vi "Dictionary Open Object Reference__ogtk.vi"(8 "error in (no error)":errorcluster) -> (0 "error out":errorcluster, 3 "Object RefNum":T1)   [LabVIEW 2017]
uses:
  <userlib>/_OpenG.lib/dictionary/dictionary.llb/Dictionary Object RefNum__ogtk.ctl
  <userlib>/_OpenG.lib/dictionary/dictionary.llb/Dictionary Object RefNum - Enum__ogtk.ctl
  <userlib>/_OpenG.lib/dictionary/dictionary.llb/Dictionary Object Data Core Task Enum__ogtk.ctl
panel:
  # "<VI Name>\n\n<VI Description>\n\nPlease visit http://www.OpenG.org to learn about the\nOpen Source LabVIEW software movement.\n\nNOTICE -- YOU MUST LEAVE THIS NOTICE IN PLACE.  PER THE TERMS OF THE LICENSE BELOW, YOU MAY SUBLICENSE THIS SOFTWARE \nIN ANY WAY THAT DOES NOT CONFLICT WITH THIS LICENSE.\n\n### BSD License (http://www.opensource.org/licenses/bsd-license.php) Begin ###\n \nCopyright (c) 2003, Jim Kring <jim@jimkring.com>\n\nAll rights reserved.\n\nRedistribution and use in source and binary forms, with or without modification, are permitted provided that the following conditions are met:\n\n    * Redistributions of source code must retain the above copyright notice, this list of conditions and the following disclaimer.\n    * Redistributions in binary form must reproduce the above copyright notice, this list of conditions and the following disclaimer in the \n       documentation and/or other materials provided with the distribution.\n    * Neither the name of SciWare, James Kring, Inc., nor the names of its contributors may be used to endorse or promote products derived \n       from this software without specific prior written permission.\n\nTHIS SOFTWARE IS PROVIDED BY THE COPYRIGHT HOLDERS AND CONTRIBUTORS \"AS IS\" AND ANY EXPRESS OR IMPLIED WARRANTIES, \nINCLUDING, BUT NOT LIMITED TO, THE IMPLIED WARRANTIES OF MERCHANTABILITY AND FITNESS FOR A PARTICULAR PURPOSE ARE \nDISCLAIMED. IN NO EVENT SHALL THE COPYRIGHT OWNER OR CONTRIBUTORS BE LIABLE FOR ANY DIRECT, INDIRECT, INCIDENTAL,\n SPECIAL, EXEMPLARY, OR CONSEQUENTIAL DAMAGES (INCLUDING, BUT NOT LIMITED TO, PROCUREMENT OF SUBSTITUTE GOODS OR \nSERVICES; LOSS OF USE, DATA, OR PROFITS; OR BUSINESS INTERRUPTION) HOWEVER CAUSED AND ON ANY THEORY OF LIABILITY, \nWHETHER IN CONTRACT, STRICT LIABILITY, OR TORT (INCLUDING NEGLIGENCE OR OTHERWISE) ARISING IN ANY WAY OUT OF THE USE \nOF THIS SOFTWARE, EVEN IF ADVISED OF THE POSSIBILITY OF SUCH DAMAGE.\n\n### BSD License End ###"
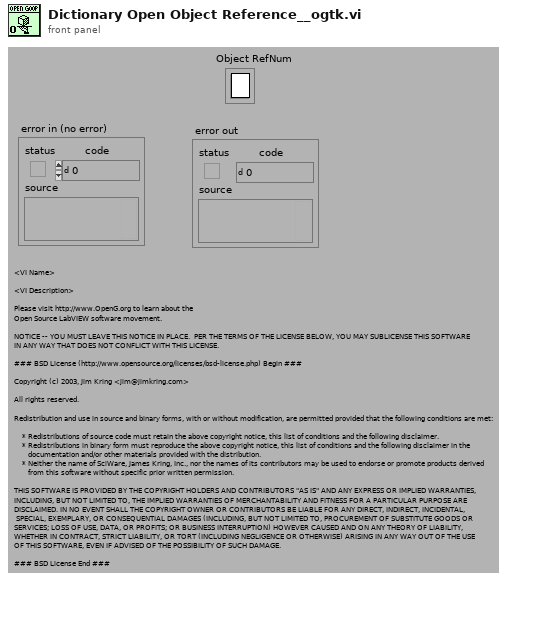
[diagram p1: front panel]
types:
  T1 = typedef "Dictionary Object RefNum__ogtk.ctl" = refnum<k1>
  T2 = typedef "Dictionary Object Data Core Task Enum__ogtk.ctl" = enum16{"read", "write", "init"}
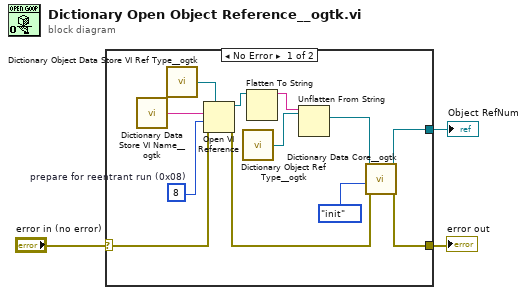
[diagram p0: block diagram]
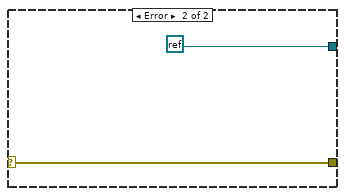
[diagram p2: hidden frame]
diagram:
  n1 = case shown="No Error" "error in (no error)" {
    selector: "error in (no error)" -> [w4 w17]
    tunnel: [w7 refnum<k0> refnum] -> w3
    tunnel: [w6 w17] -> w2
    frame No Error {
      w15 = 8  # prepare for reentrant run (0x08)
      n2 = call <userlib>:"Dictionary Data Store VI Name__ogtk.vi"() -> ("Data Store VI Name"=w5:string)
      n3 = call <userlib>:"Dictionary Object Data Store VI Ref Type__ogtk.vi"() -> ("VI Refnum (Object Data Store.vi Type)"=w14:refnum<vi>)  [unwired: 5 in]
      n4 = Open VI Reference(type specifier VI Refnum (for type only)=w14, vi path=w5, options=w15, error in (no error)=w4) -> (vi reference=w13:refnum<vi>, error out=w8:errorcluster)  [unwired: 2 in]
      n5 = call <userlib>:"Dictionary Object Ref Type__ogtk.vi"() -> ("Object RefNum Type"=w12:T1)  [unwired: 5 in]
      n6 = Flatten To String(anything=w13) -> (data string=w11:string)  [unwired: 3 in, 2 out]
      n7 = Unflatten From String(type=w12, binary string=w11) -> (value=w10:T1)  [unwired: 3 in, 2 out]
      n8 = call <userlib>:"Dictionary Data Core__ogtk.vi"("error in (no error)"=w8, "task (read)"=Dictionary_Object_Data_Core_Task_Enum__ogtk."init", "Object RefNum"=w10) -> ("error out"=w6:errorcluster, "dup Object RefNum"=w7:T1)  [unwired: 6 in, 1 out]
    }
    frame Error {
    }
  }
  "error out" <- w2
  "Object RefNum" <- w3
